vi "2_Calculate according to Expression_solution.vi"(11 "x":i32) -> (3 "Y":i32)   [LabVIEW 2014]
panel:
  # "Calculate Y according to the following expression"
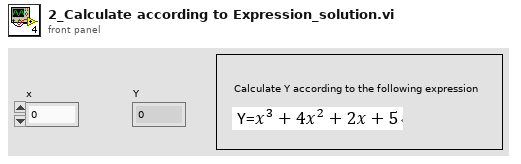
[diagram p1: front panel]
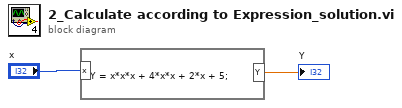
[diagram p0: block diagram]
diagram:
  n1 = formula code="Y = x*x*x + 4*x*x + 2*x + 5;"("x"="x") -> ("Y"=→"Y":dbl)
